vi "Get Target Name by PID.vi"(10 "Full Name?":bool, 11 "Device Model":u32) -> (2 "Article":string, 3 "Device Model Str":string)   [LabVIEW 2021]
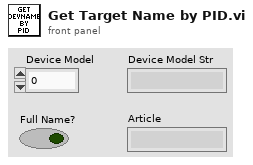
[diagram p1: front panel]
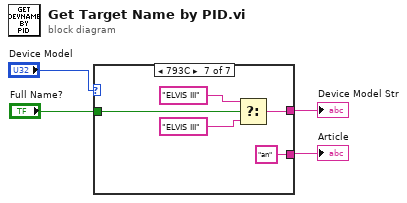
[diagram p0: block diagram]
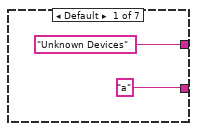
[diagram p2: hidden frame]
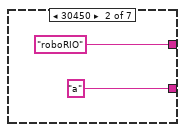
[diagram p3: hidden frame]
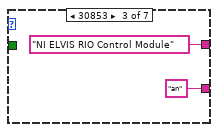
[diagram p4: hidden frame]
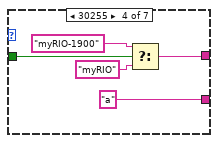
[diagram p5: hidden frame]
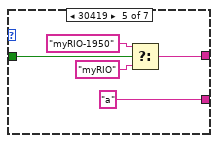
[diagram p6: hidden frame]
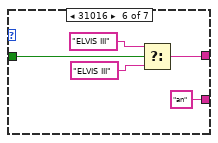
[diagram p7: hidden frame]
diagram:
  n1 = case shown="793C" "Device Model" {
    tunnel: ["Unknown Devices" "roboRIO" "NI ELVIS RIO Control Module" w12 w17 w23 w27] -> w3
    tunnel: "Full Name?" -> [_ _ _ w14 w20 w21 w26]
    tunnel: ["a" "a" "an" "a" "a" "an" "an"] -> w1
    frame Default {
    }
    frame 30450 {
    }
    frame 30853 {
    }
    frame 30255 {
      n2 = Select(t="myRIO-1900", s=w14, f="myRIO") -> (s? t:f=w12:string)
    }
    frame 30419 {
      n3 = Select(t="myRIO-1950", s=w20, f="myRIO") -> (s? t:f=w17:string)
    }
    frame 31016 {
      n4 = Select(t="ELVIS III", s=w21, f="ELVIS III") -> (s? t:f=w23:string)
    }
    frame 31036 {
      n5 = Select(t="ELVIS III", s=w26, f="ELVIS III") -> (s? t:f=w27:string)
    }
  }
  "Device Model Str" <- w3
  "Article" <- w1
